vi "Module Data - Append Newly Handled Error.vi"(2 "Index of the newly reported error in the OSI data structure":i32, 3 "Newly Reported Error":T8, 4 "Module Data in":T3) -> (0 "Error to be logged":T1, 1 "Module Data out (Error appended)":T3)   [LabVIEW 2023, in "Error Manager.lvlib"]
doc: "Blank VI with error handling."
uses:
  Error Manager.lvlib
  Module Data (cluster).ctl
  Handled Error (cluster).ctl
  Read-Unread Status (enum).ctl
  Display Order (enum).ctl
  Error in current one-second interval (cluster).ctl
  Reported Error (cluster).ctl
  Pop-up New Error Dialogue Instruction (enum).ctl
  Error Log/Error to be logged (cluster).ctl
  Error Log/Error Type (enum).ctl
  Error Log/ErrorLog.lvlib
panel:
  out "Total no. of errors logged so far":i32
  # "Input\nInputs to the VI"
  # "Development\nControls or indicators that are useful for development or testing, but which are not outputs of the VI."
  # "Output\nOutputs of the VI"
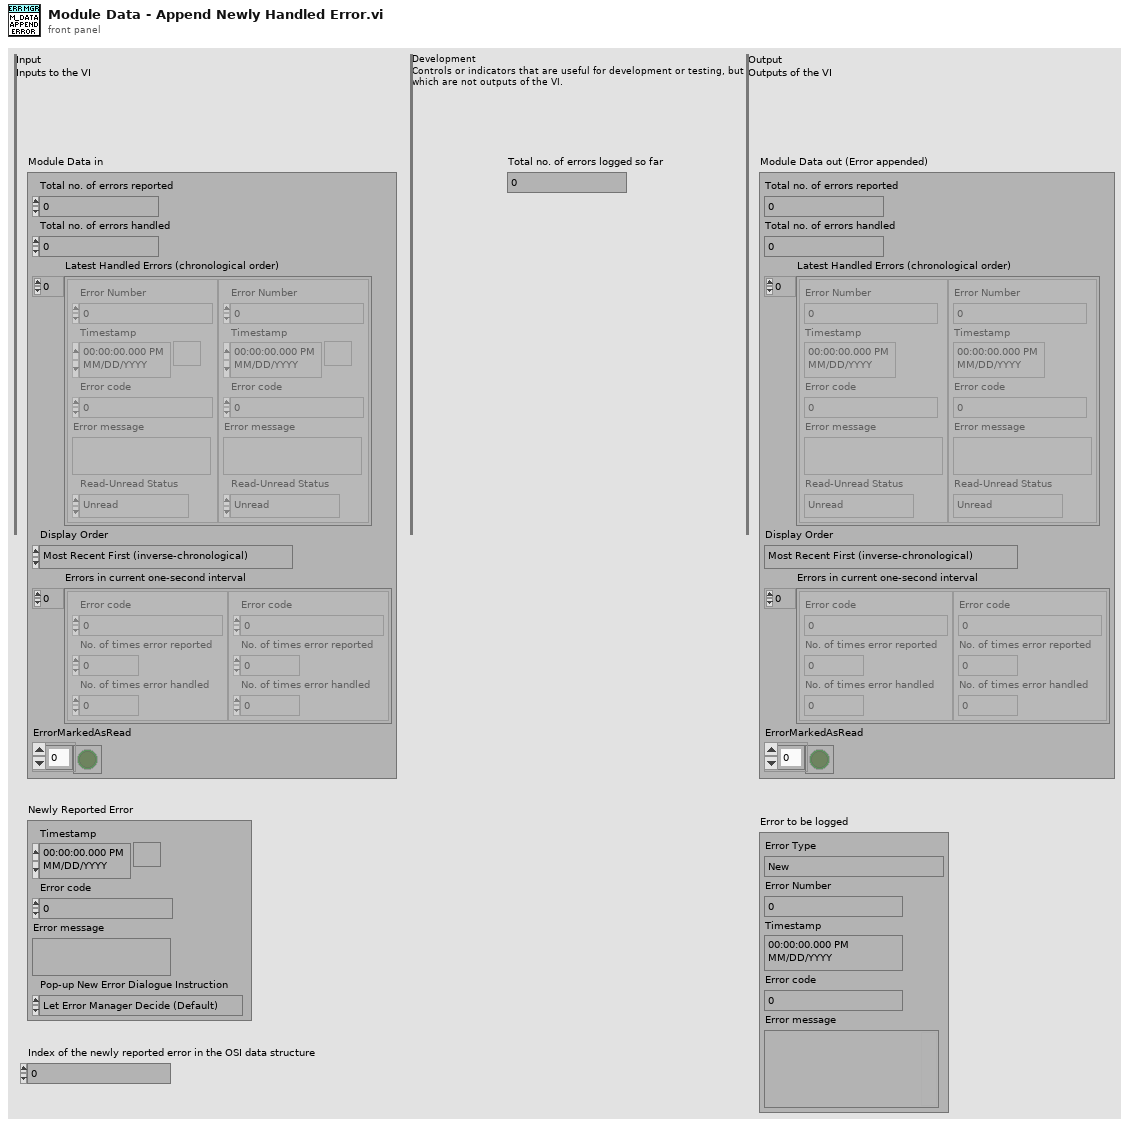
[diagram p1: front panel]
types:
  T1 = typedef "Error Manager.lvlib/ErrorLog.lvlib/Error to be logged (cluster).ctl" = cluster{"Error Type":T2, "Error Number":i32, "Timestamp":timestamp, "Error code":i32, "Error message":string}
  T2 = typedef "Error Manager.lvlib/ErrorLog.lvlib/Error Type (enum).ctl" = enum16{"New", "Identical to last logged error"}
  T3 = typedef "Error Manager.lvlib/Module Data (cluster).ctl" = cluster{"Total no. of errors reported":i32, "Total no. of errors handled":i32, "Latest Handled Errors (chronological order)":T4[], "Display Order":T6, "Errors in current one-second interval":T7[], "ErrorMarkedAsRead":bool[]}
  T4 = typedef "Error Manager.lvlib/Handled Error (cluster).ctl" = cluster{"Error Number":i32, "Timestamp":timestamp, "Error code":i32, "Error message":string, "Read-Unread Status":T5}
  T5 = typedef "Error Manager.lvlib/Read-Unread Status (enum).ctl" = enum16{"Unread", "Read"}
  T6 = typedef "Error Manager.lvlib/Display Order (enum).ctl" = enum16{"Most Recent First (inverse-chronological)", "Oldest First (chronological)"}
  T7 = typedef "Error Manager.lvlib/Error in current one-second interval (cluster).ctl" = cluster{"Error code":i32, "No. of times error reported":u32, "No. of times error handled":u32}
  T8 = typedef "Error Manager.lvlib/Reported Error (cluster).ctl" = cluster{"Timestamp":timestamp, "Error code":i32, "Error message":string, "Pop-up New Error Dialogue Instruction":T9}
  T9 = typedef "Error Manager.lvlib/Pop-up New Error Dialogue Instruction (enum).ctl" = enum16{"Let Error Manager Decide (Default)", "Don't pop-up", "Pop-up"}
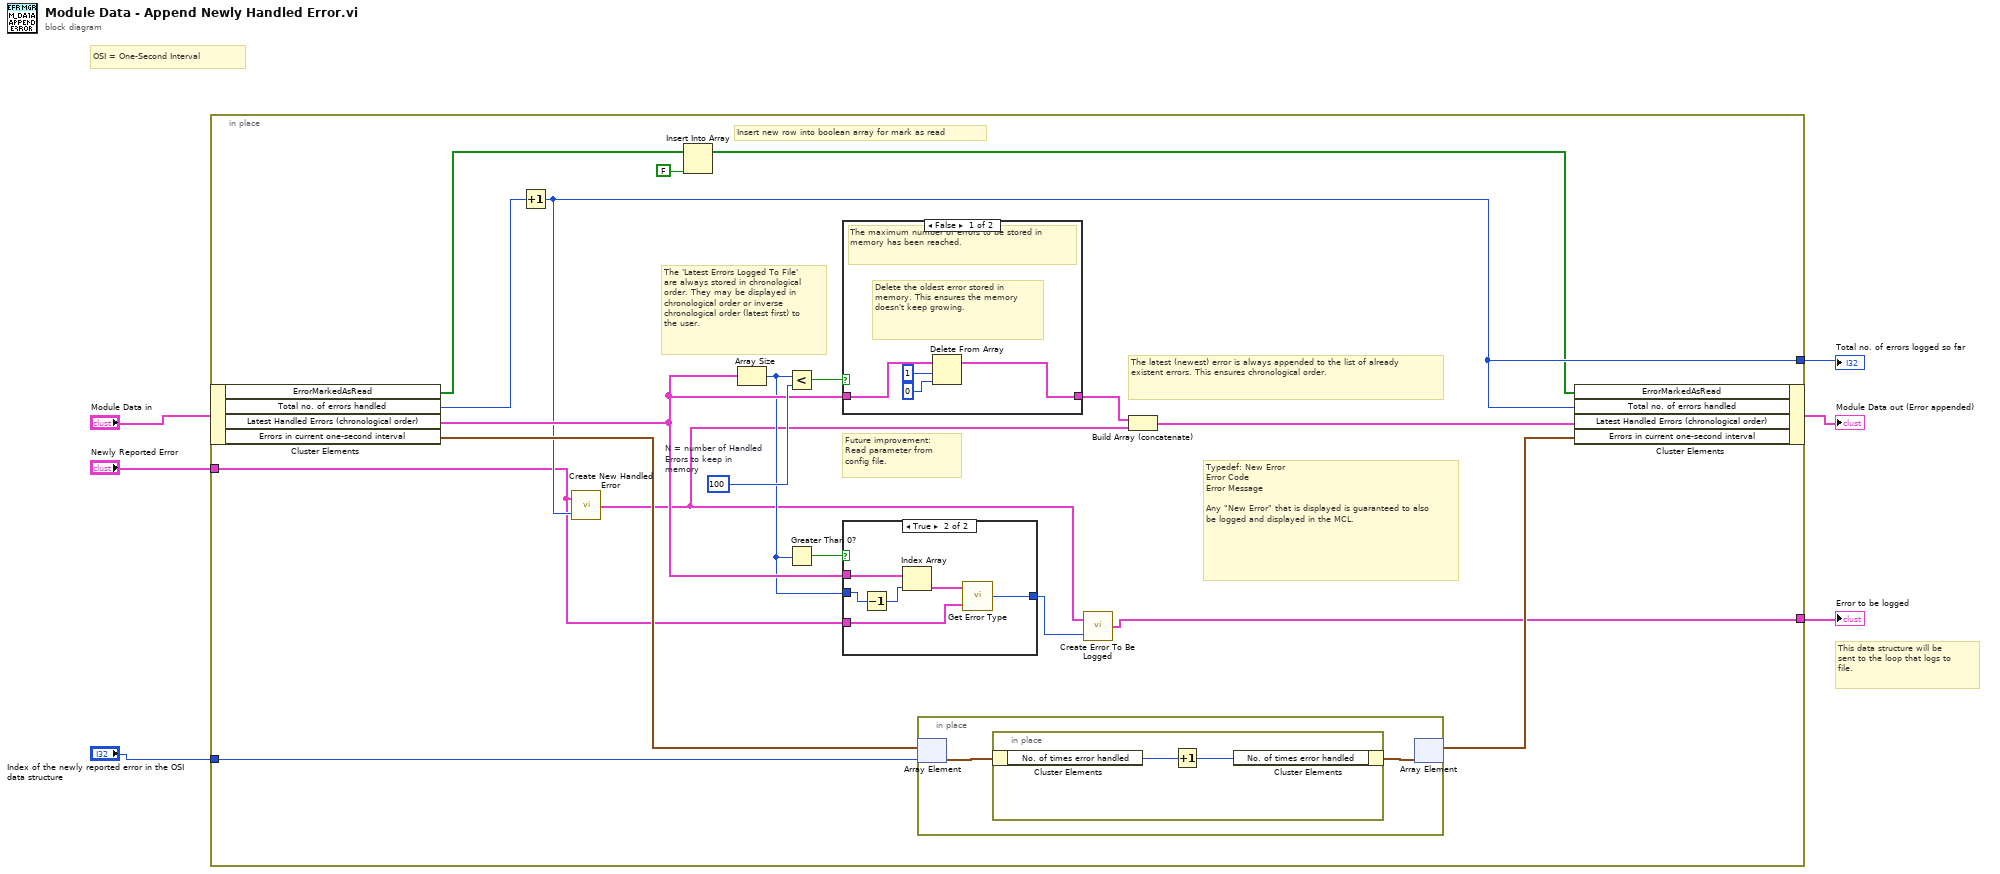
[diagram p0: block diagram]
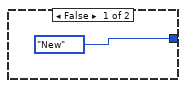
[diagram p2: hidden frame]
diagram:
  # "This data structure will be sent to the loop that logs to file."
  # "OSI = One-Second Interval"
  n1 = in-place {
    in-place-border: "Newly Reported Error" -> [w13]
    in-place-border: [w14] -> w2
    in-place-border: "Index of the newly reported error in the OSI data structure" -> [w23]
    in-place-border: [w11] -> w1
    w21 = 100  # N = number of Handled Errors to keep in memory
    # "Typedef: New Error\nError Code\nError Message\n\nAny \"New Error\" that is displayed is guaranteed to also be logged and displayed in the MCL."
    # "Insert new row into boolean array for mark as read"
    # "Future improvement: Read parameter from config file."
    # "The 'Latest Errors Logged To File' are always stored in chronological order. They may be displayed in chronological order or inverse chronological order (latest first) to the user."
    # "The latest (newest) error is always appended to the list of already existent errors. This ensures chronological order."
    n2 = in-place-cluster #1("Module Data in") -> ("ErrorMarkedAsRead"=w9:bool[], "Total no. of errors handled"=w18:i32, "Latest Handled Errors (chronological order)"=w16:T4[], "Errors in current one-second interval"=w24:T7[])
    n3 = Increment(x=w18) -> (x+1=w14:i32)
    n4 = call "Create New Handled Error.vi"("Error Number"=w14, "Reported Error"=w13) -> ("Handled Error"=w10:T4)
    n5 = Insert Into Array(array=w9, new element=FALSE) -> (w7:bool[])  [unwired: 1 in]
    n6 = Array Size(array=w16) -> (size(s)=w15:i32)
    n7 = Less?(x=w15, y=w21) -> (x < y?=w20:bool)
    n8 = Greater Than 0?(x=w15) -> (x > 0?=w17:bool)
    n9 = case shown="False" w20 {
      tunnel: w16 -> [w36 w37]
      tunnel: [w33 w37] -> w19
      frame False {
        # "Delete the oldest error stored in memory. This ensures the memory doesn't keep growing."
        # "The maximum number of errors to be stored in memory has been reached."
        n10 = Delete From Array(array=w36, length=1, index=0) -> (array with subset deleted=w33:T4[])  [unwired: 1 out]
      }
      frame True {
      }
    }
    n11 = case shown="True" w17 {
      tunnel: [Error_Type_(enum)."New" ("Error Type") w27] -> w12
      tunnel: w16 -> [_ w32]
      tunnel: w15 -> [_ w31]
      tunnel: w13 -> [_ w28]
      frame False {
      }
      frame True {
        n12 = Decrement(x=w31) -> (x-1=w30:i32)
        n13 = Index Array(array=w32, index=w30) -> (element=w29:T4)
        n14 = call "Get Error Type.vi"("Newly Reported Error"=w28, "Last (latest) Handled Error"=w29) -> ("Error Type"=w27:T2)
      }
    }
    n15 = in-place {
      n16 = in-place-array #2(w24, w23) -> (w39:T7)
      n17 = in-place {
        n18 = in-place-cluster #3(w39) -> ("No. of times error handled"=w41:u32)
        n19 = Increment(x=w41) -> (x+1=w40:u32)
        n20 = in-place-cluster #3("No. of times error handled"=w40) -> (w38:T7)
      }
      n21 = in-place-array #2(w38) -> (w22:T7[])  [unwired: 1 out]
    }
    n22 = call "Create Error To Be Logged.vi"("Error Type"=w12, "Handled Error"=w10) -> ("Error to be logged"=w11:T1)
    n23 = Build Array (concatenate)(w19, w10) -> (w25:T4[])
    n24 = in-place-cluster #1("ErrorMarkedAsRead"=w7, "Total no. of errors handled"=w14, "Latest Handled Errors (chronological order)"=w25, "Errors in current one-second interval"=w22) -> (→"Module Data out (Error appended)":T3)
  }
  "Total no. of errors logged so far" <- w2
  "Error to be logged" <- w1
